vi "Set Inline Buffer.vi"(8 "error in (no error)":errorcluster, 10 "base Inline Buffer":refnum<class "Buffer.lvclass">, 11 "Data Server Thread in":refnum<class "Data Server Thread.lvclass">) -> (0 "error out":errorcluster, 3 "Data Server Thread out":refnum<class "Data Server Thread.lvclass">)   [LabVIEW 2017, in "DSF Core.lvlib" / "Data Server Thread.lvclass"]
uses:
  Data Server Thread.lvclass
  Transfer/Transfer.lvclass
  Buffers/Buffers.lvclass
  Buffer/Buffer.lvclass
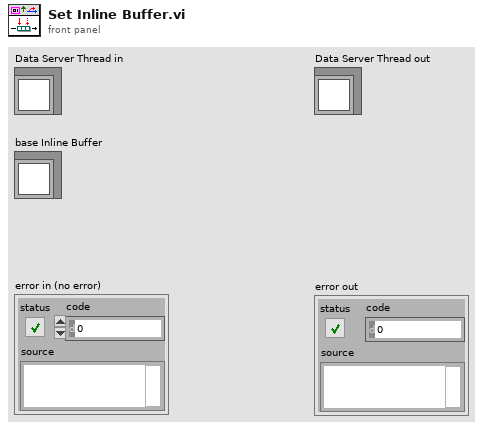
[diagram p1: front panel]
types:
  T1 = typedef "DSF Core.lvlib/Data Server Thread.lvclass/Plugin.ctl" = cluster{"Plugin Buffers":refnum<class "Buffers.lvclass">, "Plugin Status":refnum<class "Status Pointer.lvclass">, "Groups":T2[]}
  T2 = typedef "DSF Core.lvlib/Data Server Thread.lvclass/Group.ctl" = cluster{"Group Buffers":refnum<class "Buffers.lvclass">, "Group Status":refnum<class "Status Pointer.lvclass">, "Transfers":refnum<class "Transfer.lvclass">[]}
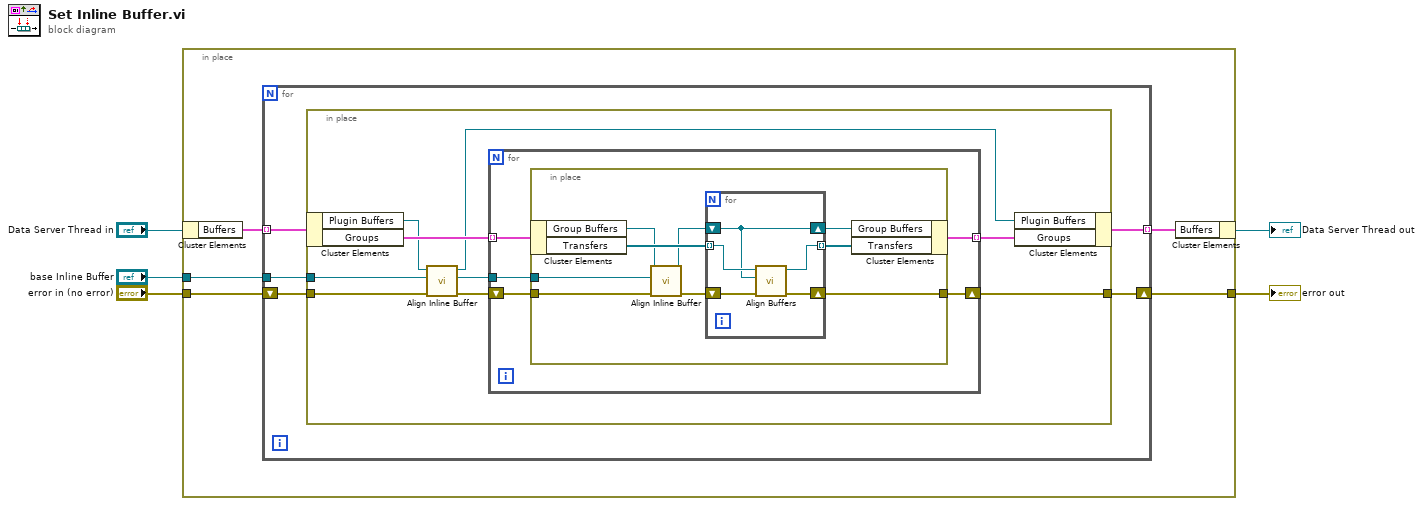
[diagram p0: block diagram]
diagram:
  n1 = in-place {
    in-place-border: "base Inline Buffer" -> [w9]
    in-place-border: "error in (no error)" -> [w8]
    in-place-border: [w7] -> w1
    n2 = in-place-cluster #1("Data Server Thread in") -> ("Buffers"=w10:T1[])
    n3 = for {
      tunnel: w10 -> [w12] mode=indexing
      tunnel: w9 -> [w15]
      shift-right: [w13] -> w7
      shift-left: w8 -> [w14]
      tunnel: [w11] -> w6 mode=indexing
      n4 = in-place {
        in-place-border: w15 -> [w19]
        in-place-border: w14 -> [w20]
        in-place-border: [w23] -> w13
        n5 = in-place-cluster #2(w12) -> ("Plugin Buffers"=w18:refnum<class "Buffers.lvclass">, "Groups"=w22:T2[])
        n6 = call "Align Inline Buffer.vi"("error in (no error)"=w20, "base Inline Buffer"=w19, "Buffers in"=w18) -> ("error out"=w16:errorcluster, "Buffers out"=w17:refnum<class "Buffers.lvclass">)  [unwired: 7 in]
        n7 = for {
          tunnel: w22 -> [w26] mode=indexing
          tunnel: w19 -> [w25]
          shift-right: [w27] -> w23
          shift-left: w16 -> [w28]
          tunnel: [w24] -> w21 mode=indexing
          n8 = in-place {
            in-place-border: w28 -> [w30]
            in-place-border: [w37] -> w27
            in-place-border: w25 -> [w31]
            n9 = in-place-cluster #3(w26) -> ("Group Buffers"=w33:refnum<class "Buffers.lvclass">, "Transfers"=w36:refnum<class "Transfer.lvclass">[])
            n10 = call "Align Inline Buffer.vi"("error in (no error)"=w30, "base Inline Buffer"=w31, "Buffers in"=w33) -> ("error out"=w29:errorcluster, "Buffers out"=w32:refnum<class "Buffers.lvclass">)  [unwired: 7 in]
            n11 = for {
              tunnel: w36 -> [w42] mode=indexing
              tunnel: [w39] -> w34 mode=indexing
              shift-right: [w40] -> w37
              shift-left: w29 -> [w41]
              shift-right: [w38] -> w35
              shift-left: w32 -> [w38]
              n12 = call "Align Buffers.vi"("error in (no error)"=w41, "Transfer Group Buffers"=w38, "Transfer in"=w42) -> ("error out"=w40:errorcluster, "Transfer out"=w39:refnum<class "Transfer.lvclass">)  [unwired: 7 in]
            }
            n13 = in-place-cluster #3("Group Buffers"=w35, "Transfers"=w34) -> (w24:T2)
          }
        }
        n14 = in-place-cluster #2("Plugin Buffers"=w17, "Groups"=w21) -> (w11:T1)
      }
    }
    n15 = in-place-cluster #1("Buffers"=w6) -> (→"Data Server Thread out":refnum<class "Data Server Thread.lvclass">)
  }
  "error out" <- w1
